vi "string_split.vi"(7 "separator (,)":string=",", 11 "string":string) -> (3 "strings":string[](array[string]))   [LabVIEW 2017, in "toml.lvlib"]
uses:
  toml.lvlib
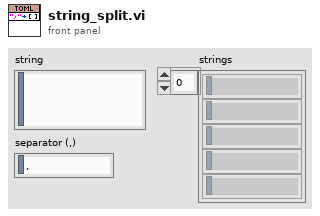
[diagram p1: front panel]
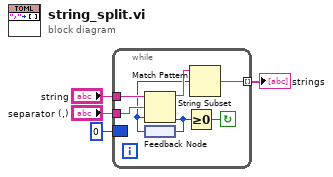
[diagram p0: block diagram]
diagram:
  n1 = while {
    tunnel: "string" -> [w11]
    tunnel: "separator (,)" -> [w10]
    tunnel: [w5] -> w2 mode=indexing
    border: 0 -> [_]
    stop <- w8 continue-if-true
    n2 = feedback #1() -> (w6:i32)
    n3 = Match Pattern(string=w11, regular expression=w10, offset (0)=w6) -> (before substring=w9:string, offset past match=w7:i32)  [unwired: 2 out]
    n4 = feedback-in #1(w7) -> ()
    n5 = Greater Or Equal To 0?(x=w7) -> (x >= 0?=w8:bool)
    n6 = String Subset(string=w9, offset (0)=w6) -> (substring=w5:string)  [unwired: 1 in]
  }
  "strings" <- w2
